vi "Update Open Node.vi"(10 "node ref in":refnum<data-value>, 11 "AD* in":refnum<class "NI_Robotics_AnytimeDStar.lvclass">) -> (2 "node ref out":refnum<data-value>, 3 "AD* out":refnum<class "NI_Robotics_AnytimeDStar.lvclass">)   [LabVIEW 2017, in "NI_Robotics_AnytimeDStar.lvclass"]
uses:
  <vilib>/robotics/Navigation/Anytime D Star/NI_Robotics_AnytimeDStar.lvclass
  <vilib>/robotics/Navigation/shared/MapNode/AbstractDstarNode/NI_Robotics_AbstractDstarNode.lvclass
  c:/Program Files (x86)/National Instruments/LabVIEW 2017/vi.lib/robotics/Navigation/shared/MapNode/AbstractMapNode/NI_Robotics_AbstractMapNode.lvclass
  <vilib>/robotics/Navigation/Anytime D Star/NI_Robotics_AnytimeDStar.lvclass/NI_Robotics_AnytimeDStar.ctl
  <vilib>/robotics/Navigation/shared/Priority Queue/NI_Robotics_Priority Queue.lvclass
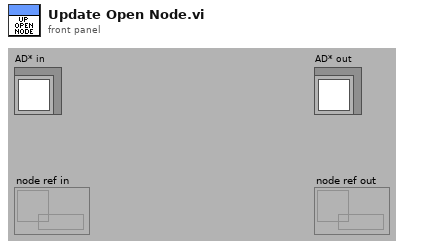
[diagram p1: front panel]
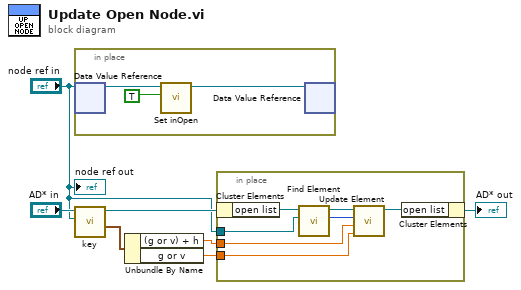
[diagram p0: block diagram]
diagram:
  n1 = in-place {
    n2 = in-place-dvr #1("node ref in") -> (w9:refnum<class "NI_Robotics_AbstractDstarNode.lvclass">)  [unwired: 1 out]
    n3 = call <vilib>:"Set inOpen.vi"("inOpen"=TRUE, "AbstractDstarNode in"=w9) -> ("AbstractDstarNode out"=w8:refnum<class "NI_Robotics_AbstractDstarNode.lvclass">)  [unwired: 8 in, 1 out]
    n4 = in-place-dvr #1(w8) -> ()  [unwired: 2 out]
  }
  n5 = call <vilib>:"key.vi"("node ref in"="node ref in", "adstar in"="AD* in") -> ("key out"=w4:cluster{"(g or v) + h":dbl, "g or v":dbl}, "adstar out"=w5:refnum<class "NI_Robotics_AnytimeDStar.lvclass">)  [unwired: 7 in, 1 out]
  n6 = Unbundle By Name(w4) -> ("(g or v) + h"=w3:dbl, "g or v"=w2:dbl)
  n7 = in-place {
    in-place-border: "node ref in" -> [w17]
    in-place-border: w3 -> [w13]
    in-place-border: w2 -> [w12]
    n8 = in-place-cluster #2(w5) -> ("open list"=w16:refnum<class "NI_Robotics_Priority Queue.lvclass">)
    n9 = call <vilib>:"Find Element.vi"("node Ref"=w17, "Priority Queue in"=w16) -> ("Numeric"=w14:i32, "Priority Queue out"=w15:refnum<class "NI_Robotics_Priority Queue.lvclass">)  [unwired: 7 in, 1 out]
    n10 = call <vilib>:"Update Element.vi"("g"=w12, "f"=w13, "index"=w14, "Priority Queue in"=w15) -> ("Priority Queue out"=w11:refnum<class "NI_Robotics_Priority Queue.lvclass">)  [unwired: 7 in]
    n11 = in-place-cluster #2("open list"=w11) -> (→"AD* out":refnum<class "NI_Robotics_AnytimeDStar.lvclass">)
  }
  "node ref out" <- "node ref in"
